vi "FTW-Endpoint-Bind.vi"(0 "FTW Endpoint":refnum<class "FTW-Endpoint.lvclass">, 5 "Endpoint Address":string, 7 "Requested Identity":string, 11 "error in":errorcluster) -> (4 "FTW Endpoint out":refnum<class "FTW-Endpoint.lvclass">, 6 "Actual Endpoint Address":string, 8 "Actual Identity":string, 15 "error out":errorcluster)   [LabVIEW 2013, in "FTW-Endpoint.lvclass"]
uses:
  FTW-Endpoint.lvclass
  FTW-Endpoint.lvclass/FTW-Endpoint.ctl
panel:
  # "Inputs"
  # "Outputs"
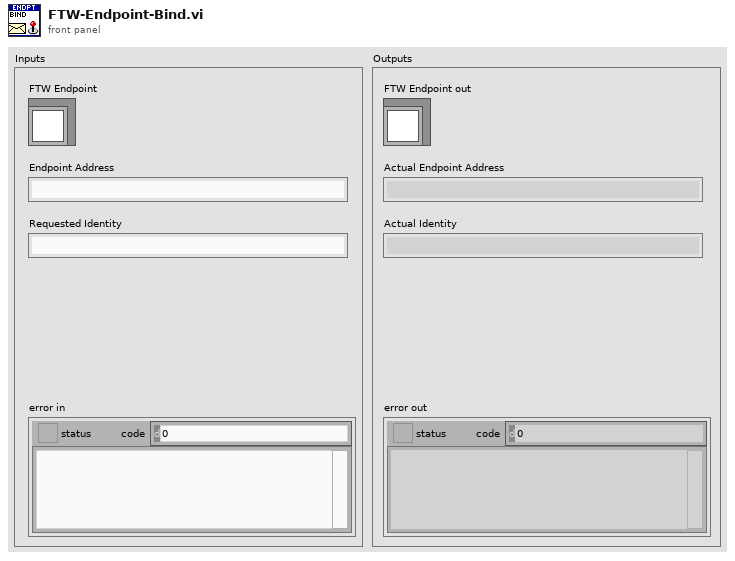
[diagram p1: front panel]
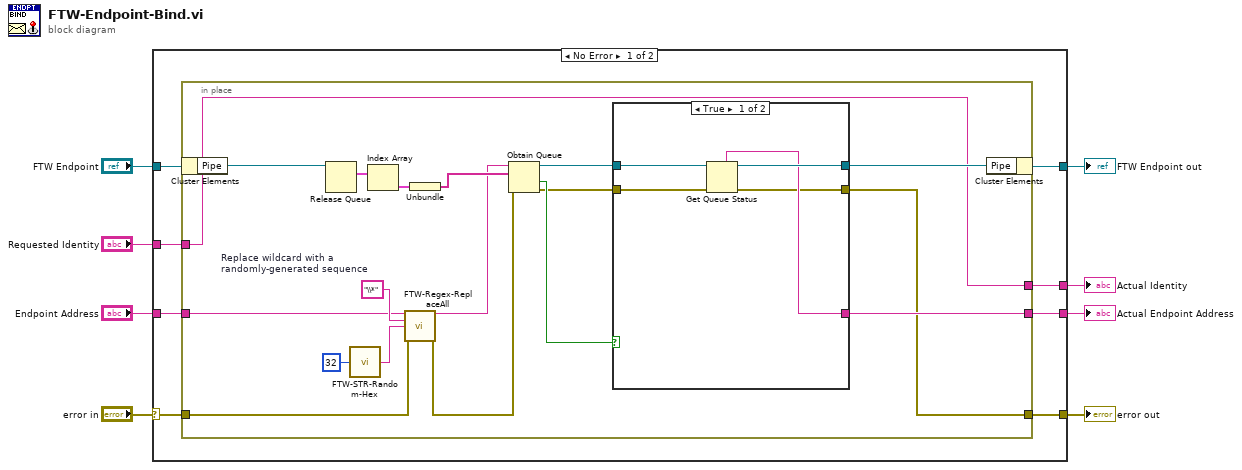
[diagram p0: block diagram]
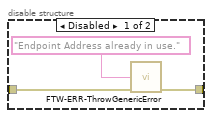
[diagram p3: hidden frame]
diagram:
  n1 = case shown="No Error" "error in" {
    selector: "error in" -> [w14 w48]
    tunnel: [w10 w48] -> w8
    tunnel: [w11 w47] -> w6
    tunnel: "FTW Endpoint" -> [w16 w47]
    tunnel: "Requested Identity" -> [w15 _]
    tunnel: "Endpoint Address" -> [w13 _]
    tunnel: [w12 _] -> w2
    tunnel: [w9 _] -> w1
    frame No Error {
      n2 = in-place {
        in-place-border: w15 -> [w24]
        in-place-border: w14 -> [w18]
        in-place-border: [w25] -> w10
        in-place-border: w13 -> [w19]
        in-place-border: [w29] -> w12
        in-place-border: [w24] -> w9
        w23 = "\\*"  # Replace wildcard with a randomly-generated sequence
        n3 = in-place-cluster #1(w16) -> ("Pipe"=w34:refnum<queue>)
        n4 = Release Queue(queue=w34) -> (remaining elements=w33:cluster{"Multipart Message":string[]}[])  [unwired: 2 in, 2 out]
        n5 = call "FTW-STR-Random-Hex.vi"("String Length"=32) -> ("Random Hex String"=w21:string)  [unwired: 3 in]
        n6 = Index Array(array=w33) -> (element=w32:cluster{"Multipart Message":string[]})  [unwired: 1 in]
        n7 = call "FTW-Regex-ReplaceAll.vi"("String"=w19, "Search for (Regular Expression)"=w23, "Replace with"=w21, "error in"=w18) -> ("String out"=w20:string, "error out"=w17:errorcluster)  [unwired: 9 in, 1 out]
        n8 = Unbundle(w32) -> ("Multipart Message"=w31:string[])
        n9 = Obtain Queue(name (unnamed)=w20, element data type=w31, error in (no error)=w17) -> (queue out=w27:refnum<queue>, created new?=w30:bool, error out=w26:errorcluster)  [unwired: 2 in]
        n10 = case shown="True" w30 {
          tunnel: [w36 _] -> w29
          tunnel: [w38 w41] -> w28
          tunnel: w27 -> [w39 w41]
          tunnel: w26 -> [w37 w42]
          tunnel: [w35 w40] -> w25
          frame True {
            n11 = Get Queue Status(queue=w39, error in (no error)=w37) -> (queue out=w38:refnum<queue>, queue name=w36:string, error out=w35:errorcluster)  [unwired: 1 in, 5 out]
          }
          frame False {
            n12 = disable-structure shown="Enabled" {
              disable-tunnel: w42 -> [w45 w46]
              disable-tunnel: [w44 w46] -> w40
              frame Disabled {
                n13 = call "FTW-ERR-ThrowGenericError.vi"("Error Message"="Endpoint Address already in use.", "error in"=w45) -> ("error out"=w44:errorcluster)  [unwired: 13 in]
              }
              frame Enabled {
              }
            }
          }
        }
        n14 = in-place-cluster #1("Pipe"=w28) -> (w11:refnum<class "FTW-Endpoint.lvclass">)
      }
    }
    frame Error {
    }
  }
  "error out" <- w8
  "FTW Endpoint out" <- w6
  "Actual Endpoint Address" <- w2
  "Actual Identity" <- w1
